vi "Function_new plot.vi"(8 "error in (no error)":errorcluster, 10 "Array in":refnum<queue>[](array[refnum]), 11 "Boolean in":refnum<vi>) -> (0 "error out":errorcluster, 3 "Array out":refnum<queue>[](array[refnum]))   [LabVIEW 2021]
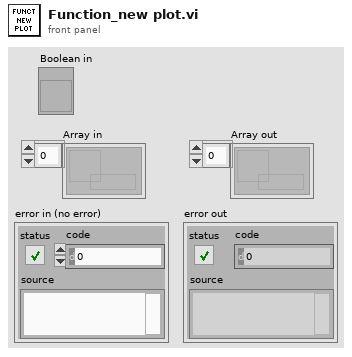
[diagram p1: front panel]
types:
  T1 = enum8{"Enabled", "Disabled", "Disabled and Grayed Out"}
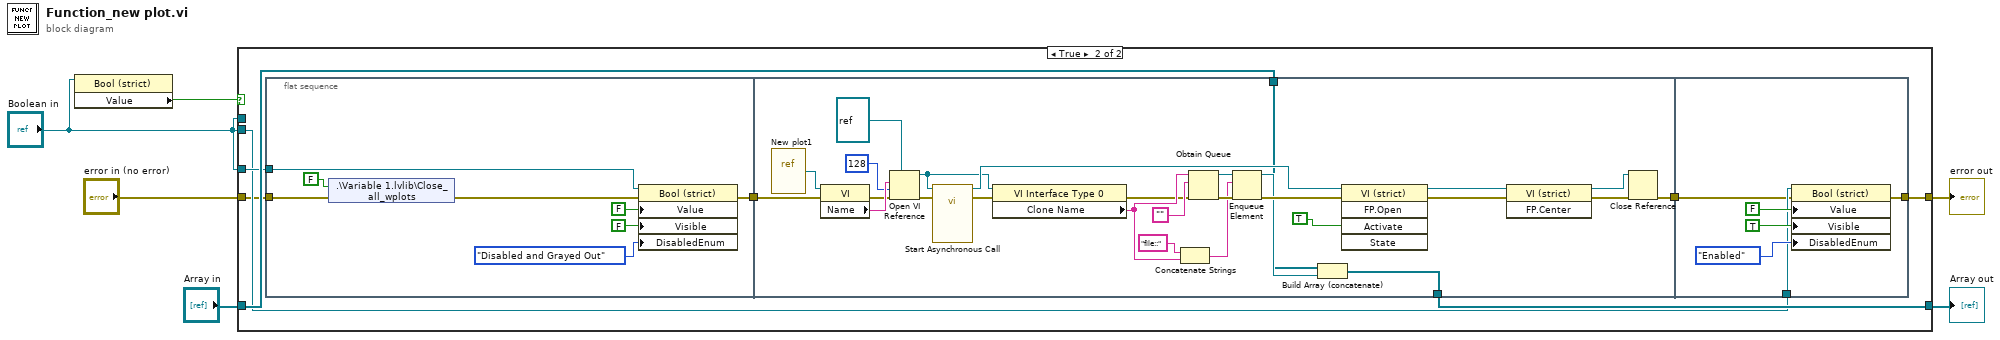
[diagram p0: block diagram]
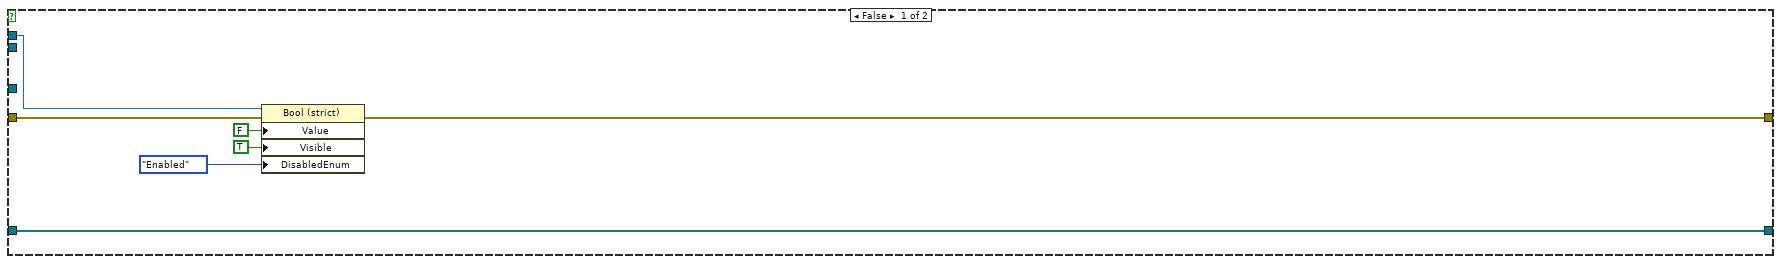
[diagram p2: hidden frame]
diagram:
  n1 = property on="Property Node" class="Bool (strict)"(reference="Boolean in") -> ("Value"=w4:bool)  [unwired: 1 in, 2 out]
  n2 = case shown="True" w4 {
    tunnel: [w10 w21] -> w5
    tunnel: "Array in" -> [w10 w20]
    tunnel: "Boolean in" -> [w9 _]
    tunnel: "Boolean in" -> [_ w19]
    tunnel: "Boolean in" -> [_ w18]
    tunnel: "error in (no error)" -> [w8 w17]
    tunnel: [w7 w14] -> w1
    frame False {
      n3 = property on="Property Node" class="Bool (strict)"(reference=w9, error in=w8, "Value"=FALSE ("New plot"), "Visible"=TRUE, "DisabledEnum"=T1."Enabled" ("Disabled")) -> (error out=w7:errorcluster)  [unwired: 1 out]
    }
    frame True {
      n4 = flat-sequence {
        tunnel: w19 -> [w24]
        tunnel: w17 -> [w23]
        tunnel: [w22] -> w16
        tunnel: [w38] -> w21
        tunnel: w20 -> [w37]
        tunnel: w16 -> [w33]
        tunnel: [w31] -> w15
        tunnel: w18 -> [w59]
        tunnel: w15 -> [w58]
        tunnel: [w57] -> w14
        frame #0 {
          n5 = shared-variable ".\\Variable 1.lvlib\\Close_all_wplots"(FALSE ("Close_all_wplots"), error in=w23) -> (error out=w25:errorcluster)
          n6 = property on="Property Node" class="Bool (strict)"(reference=w24, error in=w25, "Value"=FALSE ("New plot"), "Visible"=FALSE, "DisabledEnum"=T1."Disabled and Grayed Out" ("Disabled")) -> (error out=w22:errorcluster)  [unwired: 1 out]
        }
        frame #1 {
          n7 = vi-ref "New plot1.vi"() -> (w30:refnum<vi>)
          n8 = property class="VI"(reference=w30, error in=w33) -> (error out=w32:errorcluster, "Name"=w56:string)  [unwired: 1 out]
          n9 = Open VI Reference(type specifier VI Refnum (for type only)=refnum<vi> refnum, vi path=w56, options=128, error in (no error)=w32) -> (vi reference=w48:refnum<vi>, error out=w52:errorcluster)  [unwired: 2 in]
          n10 = call-by-ref "Start Asynchronous Call"(reference=w48, error in=w52) -> (reference out=w51:refnum<vi>, error out=w42:errorcluster)  [unwired: 2 in]
          n11 = property class="VI Interface Type 0"(reference=w48, error in=w42) -> (error out=w43:errorcluster, "Clone Name"=w45:string)  [unwired: 1 out]
          n12 = Concatenate Strings("file::" ("string"), w45) -> (w36:string)
          n13 = Obtain Queue(name (unnamed)=w45, element data type="", error in (no error)=w43) -> (queue out=w44:refnum<queue>, error out=w41:errorcluster)  [unwired: 2 in, 1 out]
          n14 = Enqueue Element(queue=w44, element=w36, error in (no error)=w41) -> (queue out=w39:refnum<queue>, error out=w40:errorcluster)  [unwired: 1 in, 1 out]
          n15 = Build Array (concatenate)(w37, w39) -> (w38:refnum<queue>[])
          n16 = invoke class="VI (strict)" method="FP.Open"(reference=w51, error in=w40, "Activate"=TRUE ("Activate?")) -> (reference out=w50:refnum<vi>, error out=w35:errorcluster)  [unwired: 2 in, 3 out]
          n17 = invoke class="VI (strict)" method="FP.Center"(reference=w50, error in=w35) -> (reference out=w49:refnum<vi>, error out=w34:errorcluster)  [unwired: 1 in, 1 out]
          n18 = Close Reference(reference=w49, error in (no error)=w34) -> (error out=w31:errorcluster)
        }
        frame #2 {
          n19 = property on="Property Node" class="Bool (strict)"(reference=w59, error in=w58, "Value"=FALSE ("Value (Signaling)"), "Visible"=TRUE, "DisabledEnum"=T1."Enabled" ("Disabled")) -> (error out=w57:errorcluster)  [unwired: 1 out]
        }
      }
    }
  }
  "Array out" <- w5
  "error out" <- w1
